vi "Test-Error Propagation.vi"   [LabVIEW 2017]
uses:
  src/Dialog Type.ctl
  <vilib>/addons/_JKI Toolkits/Caraya/classes/Assert/Assert Error.vi
  <vilib>/addons/_JKI Toolkits/Caraya/classes/Assert/Assert Not Error.vi
  <vilib>/addons/_JKI Toolkits/Caraya/classes/Test/Test.lvclass
  <vilib>/addons/_JKI Toolkits/Caraya/classes/Assert/Assert.lvclass
  src/Error Dialog w Copy to Clipboard.lvlib
types:
  T1 = typedef "Error Dialog w Copy to Clipboard.lvlib/Dialog Type.ctl" = enum16{"OK message", "Continue or Stop message"}
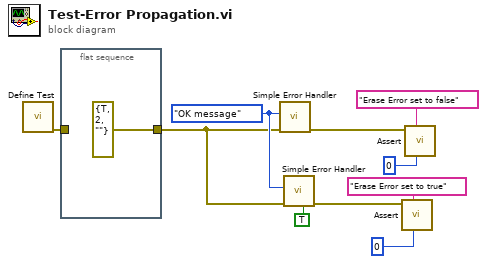
[diagram p0: block diagram]
diagram:
  w4 = Dialog_Type."OK message" ("Dialog Type")
  n1 = call <vilib>:"Define Test.vi"() -> ("error out"=w2:errorcluster)  [unwired: 11 in]
  n2 = flat-sequence {
    tunnel: w2 -> [_]
    tunnel: [errorcluster {"status"=TRUE, "code"=2, "source"=""} ("error out")] -> w1
    frame #0 {
    }
  }
  n3 = call "Simple Error Handler.vi"("error in (no error)"=w1, "Dialog Type"=w4) -> ("error out"=w8:errorcluster)  [unwired: 9 in]
  n4 = call "Simple Error Handler.vi"("Erase Error ?"=TRUE, "error in (no error)"=w1, "Dialog Type"=w4) -> ("error out"=w6:errorcluster)  [unwired: 8 in]
  n5 = call-poly <vilib>:"Assert.vi"("error code (1)"=0, "Label"="Erase Error set to true", "Not Error?"=w6) -> ()  [unwired: 8 in, 1 out]
  n6 = call-poly <vilib>:"Assert.vi"("error code (1)"=0, "Label"="Erase Error set to false", "Error?"=w8) -> ()  [unwired: 8 in, 1 out]
